vi "AlazarFFTBackgroundSubtractionGetRecordS16.vi"(4 "error in (no error)":errorcluster, 5 "Background Record In":i16[](array[numeric]), 7 "DSP Handle":u64) -> (0 "error out":errorcluster, 1 "Return Code":u32, 2 "Background Record Out":i16[](array[numeric]), 3 "DSP Handle":u64)   [LabVIEW 2009]
uses:
  ATSApi.dll
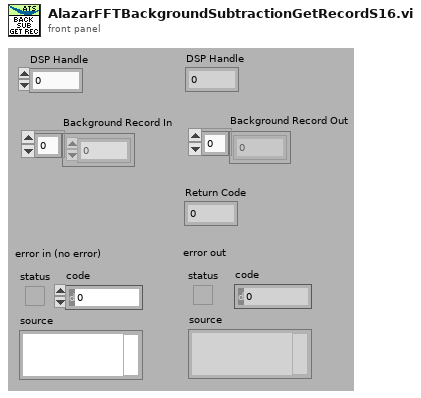
[diagram p1: front panel]
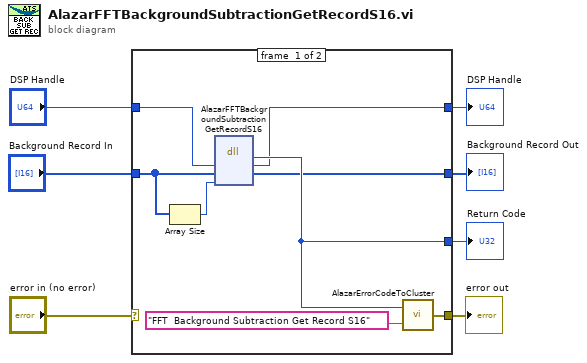
[diagram p0: block diagram]
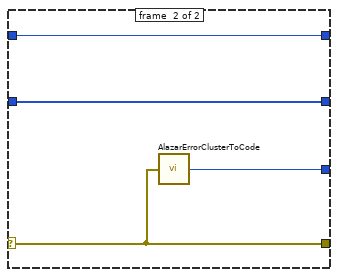
[diagram p2: hidden frame]
diagram:
  n1 = case shown="No Error" "error in (no error)" {
    selector: "error in (no error)" -> [_ w19]
    tunnel: [w12 w19] -> w6
    tunnel: [w14 w18] -> w2
    tunnel: "DSP Handle" -> [w15 w17]
    tunnel: [w11 w17] -> w4
    tunnel: "Background Record In" -> [w10 w16]
    tunnel: [w8 w16] -> w1
    frame #0 {
      n2 = Array Size(array=w10) -> (size(s)=w9:i32)
      n3 = dll-call lib="ATSApi.dll" fn="AlazarFFTBackgroundSubtractionGetRecordS16"("dspHandle"=w15, "backgroundRecord"=w10, "size_samples"=w9) -> ("return type"=w14:u32, "dspHandle"=w11:u64, "backgroundRecord"=w8:i16[])  [unwired: 4 in, 2 out]
      n4 = call "AlazarErrorCodeToCluster.vi"("Message"="FFT  Background Subtraction Get Record S16", "Error Code"=w14) -> ("error out"=w12:errorcluster)
    }
    frame #1 {
      n5 = call "AlazarErrorClusterToCode.vi"("error in (no error)"=w19) -> ("Error Code"=w18:u32)
    }
  }
  "DSP Handle" <- w4
  "error out" <- w6
  "Return Code" <- w2
  "Background Record Out" <- w1
